vi "SR830ReadCalculateAverageInputs.vi"(0 "VISA resource name":refnum<visa-resource-name>="SR830LockIn2", 3 "number of averaging points":i32=5, 5 "error in (no error)":errorcluster) -> (6 "R":dbl format="%0.3g", 7 "Temp (K)":dbl format="%0.3f", 8 "R-StDev":dbl format="%0.3g", 9 "Temp-StDev":dbl format="%0.3f", 10 "Theta (degrees)":dbl format="%0.3g", 11 "Measurement Time (s)":dbl, 12 "Theta-StDev (degrees)":dbl format="%0.3g", 13 "Measurement Bandwidth (Hz)":dbl, 14 "VISA resource name out":refnum<visa-resource-name>, 19 "error out":errorcluster)   [LabVIEW 2016]
uses:
  <vilib>/Analysis/NI_AALBase.lvlib
panel:
  # "This VI grabs input values simulatneously from the SR830, averages them anc caluclates the\nstandard deviation. The measurement time is measured and a bandwidth is calculated."
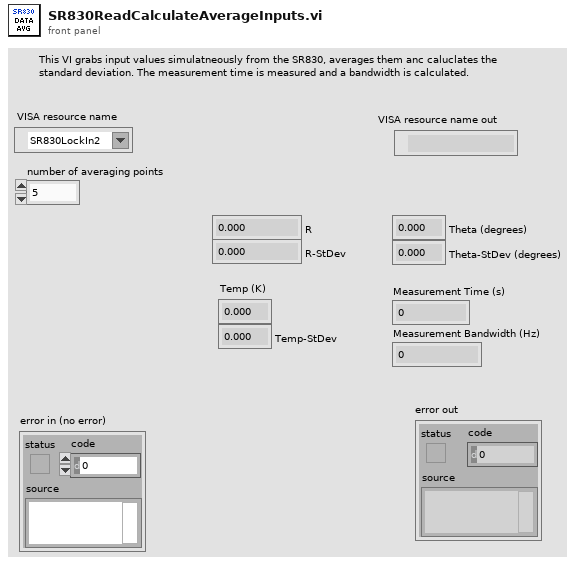
[diagram p1: front panel]
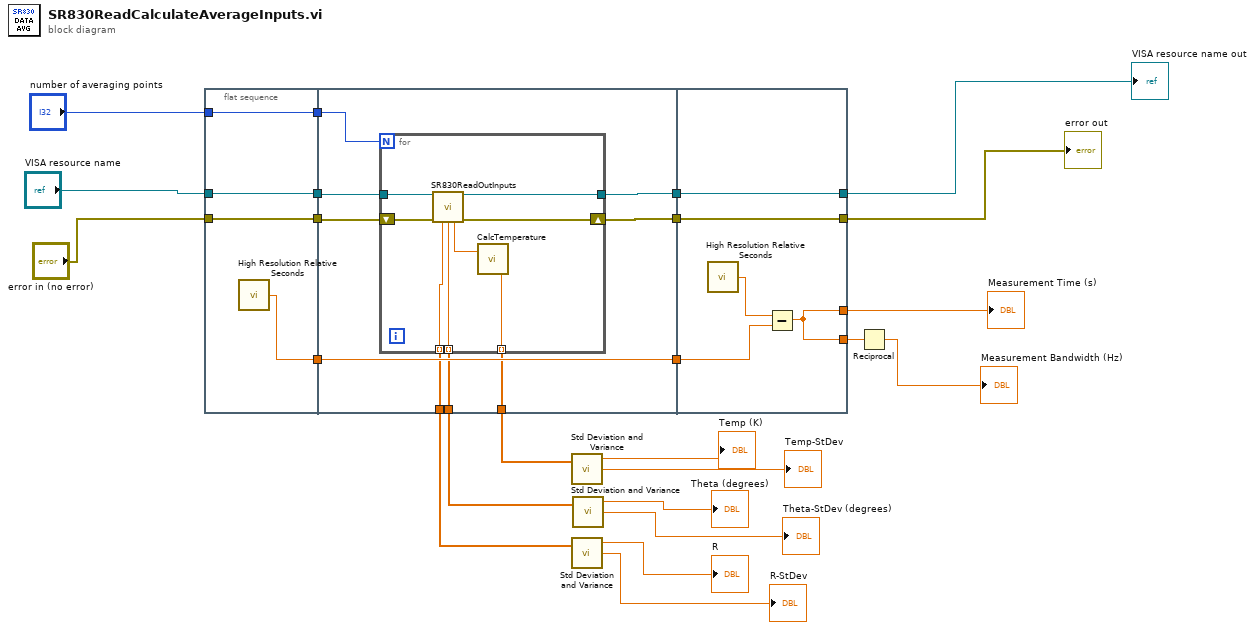
[diagram p0: block diagram]
diagram:
  n1 = flat-sequence {
    tunnel: "number of averaging points" -> [w26]
    tunnel: "error in (no error)" -> [w27]
    tunnel: "VISA resource name" -> [w28]
    tunnel: [w28] -> w19
    tunnel: [w27] -> w18
    tunnel: [w26] -> w17
    tunnel: [w25] -> w13
    tunnel: w19 -> [w37]
    tunnel: w18 -> [w36]
    tunnel: w17 -> [w35]
    tunnel: [w34] -> w16
    tunnel: [w33] -> w15
    tunnel: [w32] -> w14
    tunnel: w13 -> [w32]
    tunnel: [w31] -> w11
    tunnel: [w30] -> w9
    tunnel: [w29] -> w8
    tunnel: [w49] -> w20
    tunnel: [w50] -> w21
    tunnel: w16 -> [w50]
    tunnel: w15 -> [w49]
    tunnel: w14 -> [w47]
    tunnel: [w46] -> w12
    tunnel: [w46] -> w2
    frame #0 {
      n2 = call <vilib>:"High Resolution Relative Seconds.vi"() -> ("relative seconds"=w25:dbl)
    }
    frame #1 {
      n3 = for {
        N: w35 -> [_]
        tunnel: w37 -> [w44]
        tunnel: [w42] -> w34
        shift-right: [w41] -> w33
        shift-left: w36 -> [w43]
        tunnel: [w40] -> w31 mode=indexing
        tunnel: [w39] -> w30 mode=indexing
        tunnel: [w38] -> w29 mode=indexing
        n4 = call "SR830ReadOutInputs.vi"("VISA resource name"=w44, "error in (no error)"=w43) -> ("VISA resource name out"=w42:refnum<visa-resource-name>, "R"=w38:dbl, "Theta"=w39:dbl, "Aux In 1"=w45:dbl, "error out"=w41:errorcluster)  [unwired: 9 in]
        n5 = call "CalcTemperature.vi"("Temp Voltage (V)"=w45) -> ("Temperature (K)"=w40:dbl)  [unwired: 1 in]
      }
    }
    frame #2 {
      n6 = call <vilib>:"High Resolution Relative Seconds.vi"() -> ("relative seconds"=w48:dbl)
      n7 = Subtract(x=w48, y=w47) -> (x-y=w46:dbl)
    }
  }
  n8 = call <vilib>:"Std Deviation and Variance.vi"("X"=w11) -> ("mean"=→"Temp (K)":dbl, "standard deviation"=→"Temp-StDev":dbl)  [unwired: 1 in, 1 out]
  n9 = call <vilib>:"Std Deviation and Variance.vi"("X"=w8) -> ("mean"=→"R":dbl, "standard deviation"=→"R-StDev":dbl)  [unwired: 1 in, 1 out]
  n10 = call <vilib>:"Std Deviation and Variance.vi"("X"=w9) -> ("mean"=→"Theta (degrees)":dbl, "standard deviation"=→"Theta-StDev (degrees)":dbl)  [unwired: 1 in, 1 out]
  n11 = Reciprocal(x=w2) -> (1/x=→"Measurement Bandwidth (Hz)":dbl)
  "VISA resource name out" <- w21
  "error out" <- w20
  "Measurement Time (s)" <- w12
